vi "Serial Port - Append disconnected ports to list.vi"(8 "error in (no error)":errorcluster, 10 "Selected Values":string[](array[string]), 11 "Connected COM Ports in":string[](array[string])) -> (0 "error out":errorcluster, 3 "COM Ports out":string[](array[string]))   [LabVIEW 2011]
doc: "This VI appends the COM ports that were used last time Beagle ran to the list of connected COM ports. This is to maintain the configured values if someone has forgotten to connect the serial ports."
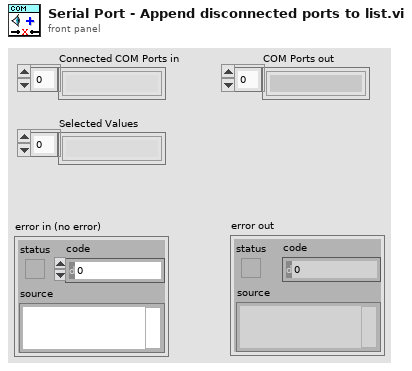
[diagram p1: front panel]
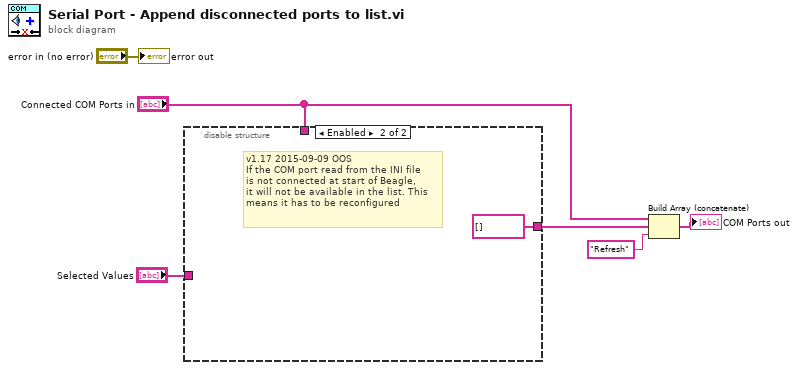
[diagram p0: block diagram]
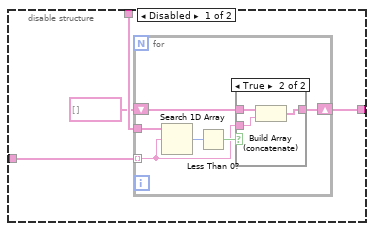
[diagram p2: hidden frame]
diagram:
  n1 = disable-structure shown="Enabled" {
    disable-tunnel: [w10 string[] []] -> w5
    disable-tunnel: "Connected COM Ports in" -> [w9 _]
    disable-tunnel: "Selected Values" -> [w7 _]
    frame Disabled {
      n2 = for {
        tunnel: w7 -> [w12] mode=indexing
        tunnel: w9 -> [w16]
        shift-right: [w13] -> w10
        shift-left: string[] [] -> [w11]
        n3 = Search 1D Array(1D array=w16, element=w12) -> (index of element=w15:i32)  [unwired: 1 in]
        n4 = Less Than 0?(x=w15) -> (x < 0?=w14:bool)
        n5 = case shown="True" w14 {
          tunnel: w12 -> [_ w18]
          tunnel: [w17 w20] -> w13
          tunnel: w11 -> [w17 w19]
          frame False {
          }
          frame True {
            n6 = Build Array (concatenate)(w19, w18) -> (w20:string[])
          }
        }
      }
    }
    frame Enabled {
      # "v1.17 2015-09-09 OOS\nIf the COM port read from the INI file\nis not connected at start of Beagle, \nit will not be available in the list. This\nmeans it has to be reconfigured"
    }
  }
  n7 = Build Array (concatenate)("Connected COM Ports in", w5, "Refresh" ("Modem Status Interface")) -> (→"COM Ports out":string[])
  "error out" <- "error in (no error)"
